vi "OR - Search for origin.vi"(8 "error in":errorcluster, 9 "Type of search":dbl format="%.2f", 10 "Axis  #":i8=1 min=1 max=6 step=1, 11 "Address / Port":i16=1 min=1 max=31 step=1) -> (0 "error out":errorcluster, 2 "Axis  # out":i8=1 min=1 max=6 step=1, 3 "Address / Port out":i16=1 min=1 max=31 step=1)   [LabVIEW 2014]
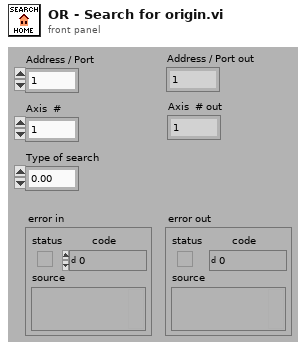
[diagram p1: front panel]
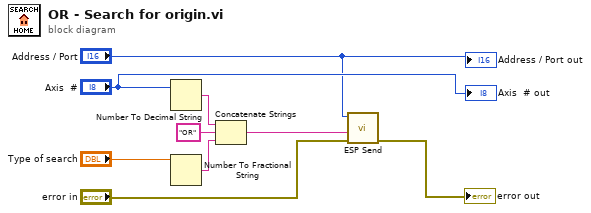
[diagram p0: block diagram]
diagram:
  n1 = Number To Decimal String(number="Axis  #") -> (decimal integer string=w8:string)  [unwired: 1 in]
  n2 = Number To Fractional String(number="Type of search") -> (F-format string=w5:string)  [unwired: 3 in]
  n3 = Concatenate Strings(w8, "OR" ("Substring"), w5) -> (w3:string)
  n4 = call "ESP Send.vi"("error in"="error in", "Command String"=w3, "Address / Port"="Address / Port") -> ("error out"=→"error out":errorcluster)  [unwired: 3 in, 1 out]
  "Address / Port out" <- "Address / Port"
  "Axis  # out" <- "Axis  #"
